vi "Parse Device Reading.vi"(8 "error in (no error)":errorcluster, 11 "Reading XML":string="<?xml version=\"1.0\" encoding=\"ISO-8859-1\" standalone=\"no\" ?>\n<methodResponse>\n\n  <params>\n    <param>\n      <value>\n        <struct>\n          <member>\n            <name>status</name>\n            <value>\n              <int>0</int>\n            </value>\n          </member>\n          <member>\n            <name>scaled</name>\n            <value>\n              <double>0.9992975666172701</double>\n            </value>\n          </member>\n          <member>\n            <name>units</name>\n            <value>Torr</value>\n          </member>\n          <member>\n            <name>name</name>\n            <value>e:201vac</value>\n          </member>\n        </struct>\n      </value>\n    </param>\n  </params>\n\n</methodResponse>\n") -> (0 "error out":errorcluster, 3 "Reading":T1)   [LabVIEW 2013]
uses:
  <vilib>/xml/Close Reference(Node).vi
  <vilib>/xml/NI_XML.lvlib
  <resource>/objmgr/DOMUserDefRef.rc
panel:
  out "Parse Errors":string
  out "XML Response":string
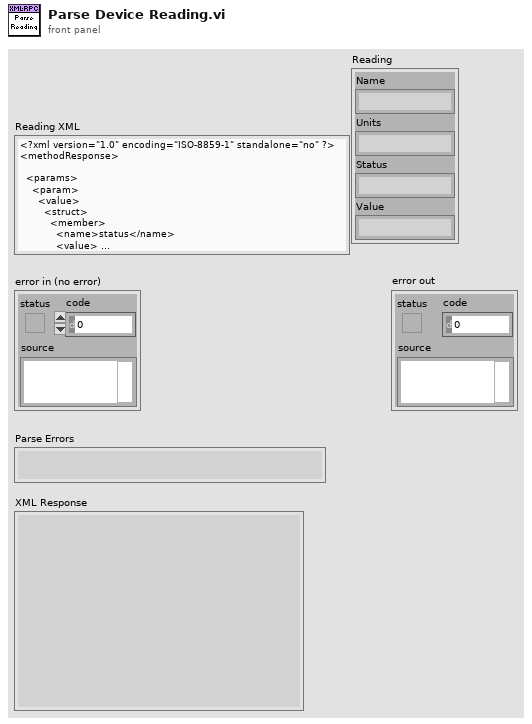
[diagram p1: front panel]
types:
  T1 = cluster{"Name":string, "Units":string, "Status":string, "Value":string}
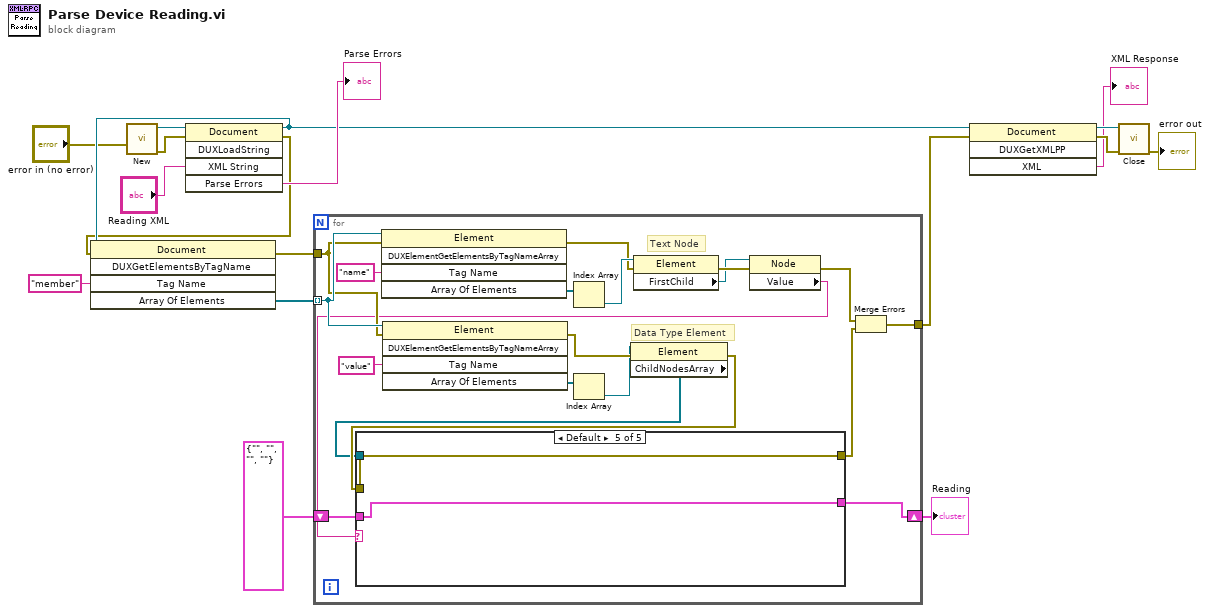
[diagram p0: block diagram]
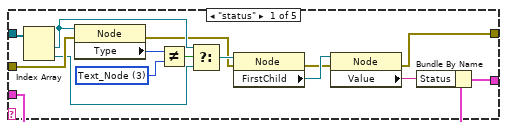
[diagram p2: hidden frame]
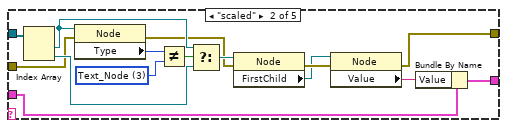
[diagram p3: hidden frame]
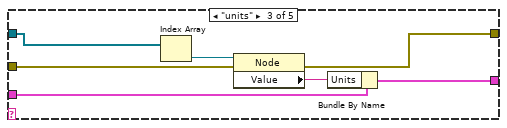
[diagram p4: hidden frame]
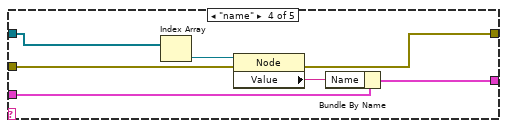
[diagram p5: hidden frame]
diagram:
  n1 = call <vilib>:"New.vi"("error in (no error)"="error in (no error)") -> ("error out"=w13:errorcluster, "DOM document out"=w12:refnum<k20>)  [unwired: 7 in]
  n2 = invoke class="Document" method="DUXLoadString"(reference=w12, error in=w13, "XML String"="Reading XML") -> (reference out=w9:refnum<k20>, error out=w8:errorcluster, "Parse Errors"=→"Parse Errors":string)  [unwired: 2 in, 2 out]
  n3 = invoke class="Document" method="DUXGetElementsByTagName"(reference=w9, error in=w8, "Tag Name"="member") -> (error out=w6:errorcluster, "Array Of Elements"=w7:refnum<k20>[])  [unwired: 2 in, 3 out]
  n4 = for {
    tunnel: w7 -> [w36] mode=indexing
    tunnel: w6 -> [w32]
    tunnel: [w25] -> w5
    shift-right: [w18] -> w1
    shift-left: T1 {"Name"="", "Units"="", "Status"="", "Value"=""} -> [w19]
    # "Data Type Element"
    # "Text Node"
    n5 = invoke class="Element" method="DUXElementGetElementsByTagNameArray"(reference=w36, error in=w32, "Tag Name"="name") -> (error out=w30:errorcluster, "Array Of Elements"=w34:refnum<k20>[])  [unwired: 2 in, 3 out]
    n6 = invoke class="Element" method="DUXElementGetElementsByTagNameArray"(reference=w36, error in=w32, "Tag Name"="value") -> (error out=w27:errorcluster, "Array Of Elements"=w33:refnum<k20>[])  [unwired: 2 in, 3 out]
    n7 = Index Array(array=w34) -> (element=w31:refnum<k20>)  [unwired: 1 in]
    n8 = Index Array(array=w33) -> (element=w22:refnum<k20>)  [unwired: 1 in]
    n9 = property class="Element"(reference=w22, error in=w27) -> (error out=w21:errorcluster, "ChildNodesArray"=w20:refnum<k20>[])  [unwired: 1 out]
    n10 = property class="Element"(reference=w31, error in=w30) -> (error out=w29:errorcluster, "FirstChild"=w28:refnum<k20>)  [unwired: 1 out]
    n11 = property class="Node"(reference=w28, error in=w29) -> (error out=w26:errorcluster, "Value"=w24:string)  [unwired: 1 out]
    n12 = case shown="Default" w24 {
      tunnel: w20 -> [w52 w59 w73 w80 _]
      tunnel: w21 -> [w48 w56 w74 w81 w83]
      tunnel: [w49 w65 w71 w78 w83] -> w23
      tunnel: w19 -> [w40 w54 w70 w77 w82]
      tunnel: [w38 w53 w68 w75 w82] -> w18
      frame "status" {
        w45 = 3 items=["Element_Node"=1, "Attribute_Node"=2, "Text_Node"=3, "CDATASection_Node"=4, "EntityReference_Node"=5, "Entity_Node"=6, "ProcessingInstruction_Node"=7, "Comment_Node"=8, "Document_Node"=9, "DocumentType_Node"=10, "DocumentFragment_Node"=11, "Notation_Node"=12] ("Node Type")
        n13 = Index Array(array=w52) -> (element #1=w44:refnum<k20>, element #2=w43:refnum<k20>)  [unwired: 2 in]
        n14 = property class="Node"(reference=w44, error in=w48) -> (error out=w41:errorcluster, "Type"=w46:i32)  [unwired: 1 out]
        n15 = Not Equal?(x=w46, y=w45) -> (x != y?=w47:bool)
        n16 = Select(t=w44, s=w47, f=w43) -> (s? t:f=w42:refnum<k20>)
        n17 = property class="Node"(reference=w42, error in=w41) -> (error out=w50:errorcluster, "FirstChild"=w51:refnum<k20>)  [unwired: 1 out]
        n18 = property class="Node"(reference=w51, error in=w50) -> (error out=w49:errorcluster, "Value"=w39:string)  [unwired: 1 out]
        n19 = Bundle By Name(cluster=w40, "Status"=w39) -> (w38:T1)
      }
      frame "scaled" {
        w62 = 3 items=["Element_Node"=1, "Attribute_Node"=2, "Text_Node"=3, "CDATASection_Node"=4, "EntityReference_Node"=5, "Entity_Node"=6, "ProcessingInstruction_Node"=7, "Comment_Node"=8, "Document_Node"=9, "DocumentType_Node"=10, "DocumentFragment_Node"=11, "Notation_Node"=12] ("Node Type")
        n20 = Index Array(array=w59) -> (element #1=w61:refnum<k20>, element #2=w60:refnum<k20>)  [unwired: 2 in]
        n21 = property class="Node"(reference=w61, error in=w56) -> (error out=w57:errorcluster, "Type"=w63:i32)  [unwired: 1 out]
        n22 = Not Equal?(x=w63, y=w62) -> (x != y?=w64:bool)
        n23 = Select(t=w61, s=w64, f=w60) -> (s? t:f=w58:refnum<k20>)
        n24 = property class="Node"(reference=w58, error in=w57) -> (error out=w67:errorcluster, "FirstChild"=w66:refnum<k20>)  [unwired: 1 out]
        n25 = property class="Node"(reference=w66, error in=w67) -> (error out=w65:errorcluster, "Value"=w55:string)  [unwired: 1 out]
        n26 = Bundle By Name(cluster=w54, "Value"=w55) -> (w53:T1)
      }
      frame "units" {
        n27 = Index Array(array=w73) -> (element=w72:refnum<k20>)  [unwired: 1 in]
        n28 = property class="Node"(reference=w72, error in=w74) -> (error out=w71:errorcluster, "Value"=w69:string)  [unwired: 1 out]
        n29 = Bundle By Name(cluster=w70, "Units"=w69) -> (w68:T1)
      }
      frame "name" {
        n30 = Index Array(array=w80) -> (element=w79:refnum<k20>)  [unwired: 1 in]
        n31 = property class="Node"(reference=w79, error in=w81) -> (error out=w78:errorcluster, "Value"=w76:string)  [unwired: 1 out]
        n32 = Bundle By Name(cluster=w77, "Name"=w76) -> (w75:T1)
      }
      frame Default {
      }
    }
    n33 = Merge Errors(w26, w23) -> (w25:errorcluster)
  }
  "Reading" <- w1
  n34 = invoke class="Document" method="DUXGetXMLPP"(reference=w9, error in=w5) -> (reference out=w16:refnum<k20>, error out=w17:errorcluster, "XML"=→"XML Response":string)  [unwired: 2 in, 1 out]
  n35 = call-poly <vilib>:"Close.vi"("error in (no error)"=w17, "node"=w16) -> ("error out"=→"error out":errorcluster)  [unwired: 7 in]
